vi "SPARK Get Device Status Warnings.vi"(8 "error in (no error)":errorcluster, 11 "MotorControlDevRef in":T2) -> (0 "error out":errorcluster, 1 "Sticky Warnings":T1, 2 "Warnings":T1, 3 "MotorControlDevRef out":T2, 4 "Timestamp":u32)   [LabVIEW 2023]
doc: "Get the active and sticky warnings of the SPARK."
uses:
  <vilib>/Rock Robotics/WPI/MotorControl/WPI_MotorControlDeviceRef.ctl
  <vilib>/Rock Robotics/WPI/MotorControl/WPI_MotorControlType.ctl
  <vilib>/Rock Robotics/SystemInterfaces/DIO/FPGA_DIOPWMChannel.ctl
  <vilib>/Rock Robotics/WPI/PWM/WPI_PWMDeadband.ctl
  <vilib>/Rock Robotics/SystemInterfaces/DIO/FPGA_DIOChannel.ctl
  Typedef/SPARK Warnings.ctl
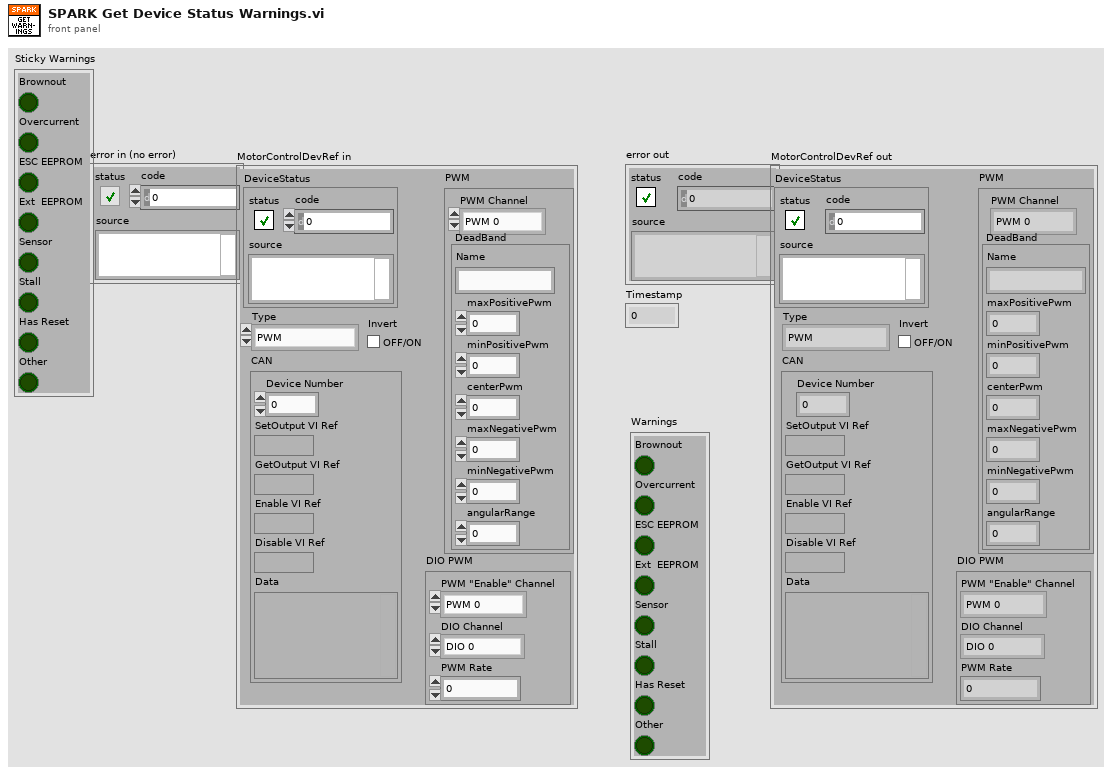
[diagram p1: front panel]
types:
  T1 = typedef "SPARK Warnings.ctl" = cluster{"Brownout":bool, "Overcurrent":bool, "ESC EEPROM":bool, "Ext  EEPROM":bool, "Sensor":bool, "Stall":bool, "Has Reset":bool, "Other":bool}
  T2 = typedef "WPI_MotorControlDeviceRef.ctl" = cluster{"DeviceStatus":errorcluster, "Type":T3, "PWM":cluster{"PWM Channel":T4, "DeadBand":T5}, "CAN":cluster{"Device Number":u8, "SetOutput VI Ref":variant, "GetOutput VI Ref":variant, "Enable VI Ref":variant, "Disable VI Ref":variant, "Data":variant}, "Invert":bool, "DIO PWM":cluster{"PWM \"Enable\" Channel":T4, "DIOChannel":T6, "PWM Rate":dbl}}
  T3 = typedef "WPI_MotorControlType.ctl" = enum16{"PWM", "CAN", "DIO PWM"}
  T4 = typedef "FPGA_DIOPWMChannel.ctl" = enum8{"PWM 0", "PWM 1", "PWM 2", "PWM 3", "PWM 4", "PWM 5", "PWM 6", "PWM 7", "PWM 8", "PWM 9", "PWM MXP 0", "PWM MXP 1", "PWM MXP 2", "PWM MXP 3", "PWM MXP 4", "PWM MXP 5", "PWM MXP 6", "PWM MXP 7", "PWM MXP 8", "PWM MXP 9", "Invalid"}
  T5 = typedef "WPI_PWMDeadband.ctl" = cluster{"Name":string, "maxPositivePwm":i32, "minPositivePwm":i32, "centerPwm":i32, "maxNegativePwm":i32, "minNegativePwm":i32, "angularRange":u16}
  T6 = typedef "FPGA_DIOChannel.ctl" = enum8{"DIO 0", "DIO 1", "DIO 2", "DIO 3", "DIO 4", "DIO 5", "DIO 6", "DIO 7", "DIO 8", "DIO 9", "DIO MXP 0", "DIO MXP 1", "DIO MXP 2", "DIO MXP 3", "DIO MXP 4", "DIO MXP 5", "DIO MXP 6", "DIO MXP 7", "DIO MXP 8", "DIO MXP 9", "DIO MXP 10", "DIO MXP 11", "DIO MXP 12", "DIO MXP 13", "DIO MXP 14", "DIO MXP 15", "SPI Port CS1", "SPI Port CS2", "SPI Port CS3", "SPI Port MISO", "SPI Port MOSI", "Invalid"}
  T7 = typedef "SPARK Status 1 Frame.ctl" = cluster{"Faults":T8, "Sticky Faults":T8, "Warnings":T1, "Sticky Warnings":T1, "Is Follower":bool, "Timestamp":u32}
  T8 = typedef "SPARK Faults.ctl" = cluster{"Other":bool, "Motor Type":bool, "Sensor":bool, "CAN":bool, "Temperature":bool, "Gate Driver":bool, "ESC EEPROM":bool, "Firmware":bool}
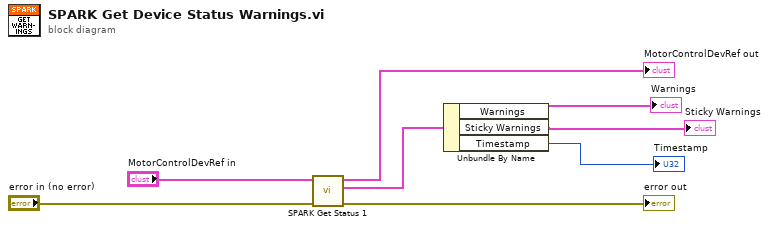
[diagram p0: block diagram]
diagram:
  n1 = call "SPARK Get Status 1.vi"("error in (no error)"="error in (no error)", "MotorControlDevRef"="MotorControlDevRef in") -> ("error out"=→"error out":errorcluster, "Status 1"=w5:T7, "MotorControlDevRef"=→"MotorControlDevRef out":T2)  [unwired: 7 in]
  n2 = Unbundle By Name(w5) -> ("Warnings"=→"Warnings":T1, "Sticky Warnings"=→"Sticky Warnings":T1, "Timestamp"=→"Timestamp":u32)
